vi "NACA0015_Polar.vi"() -> ()   [LabVIEW 2022 SP3]
panel:
  out "appended path":path
  in  "Stop Button":bool
  in  "Results folder":path
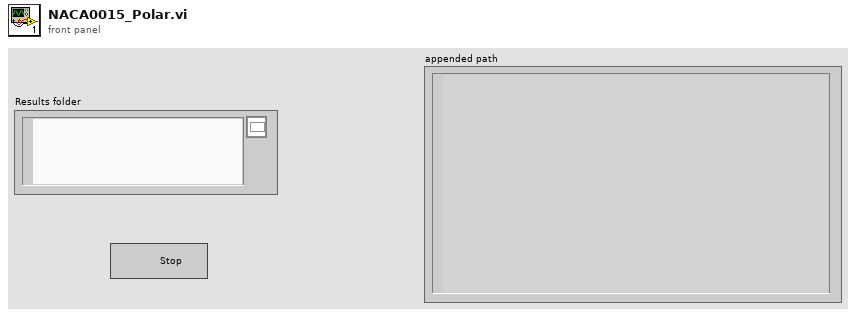
[diagram p1: front panel]
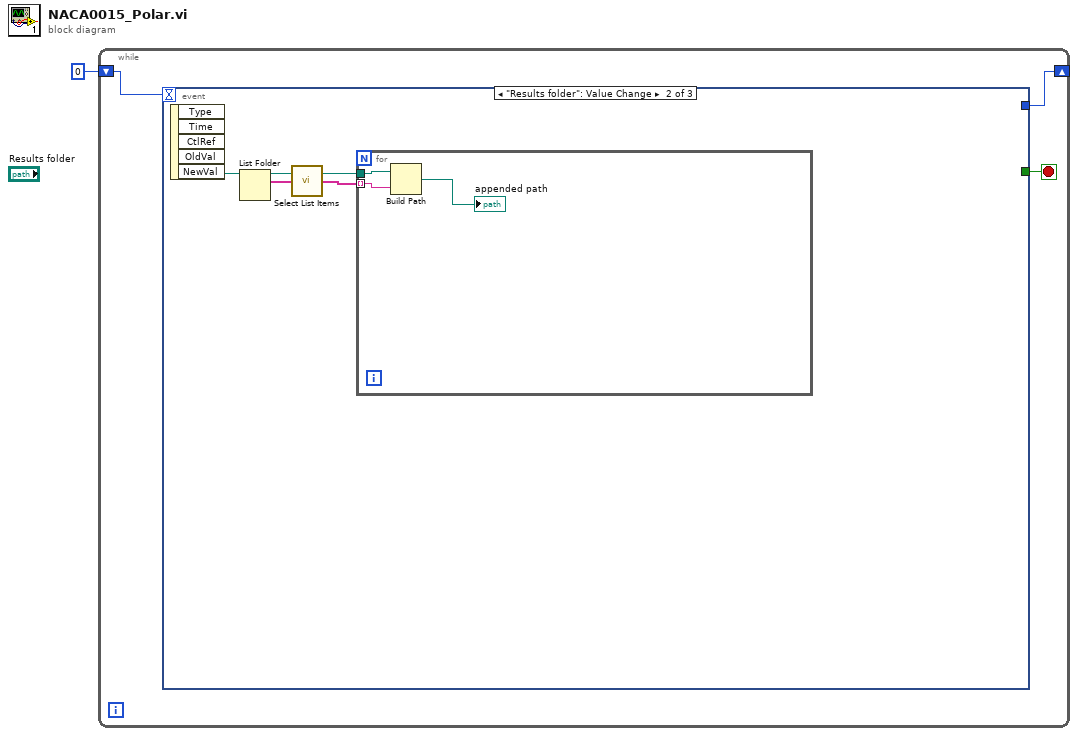
[diagram p0: block diagram]
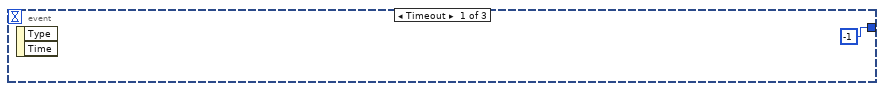
[diagram p2: hidden frame]
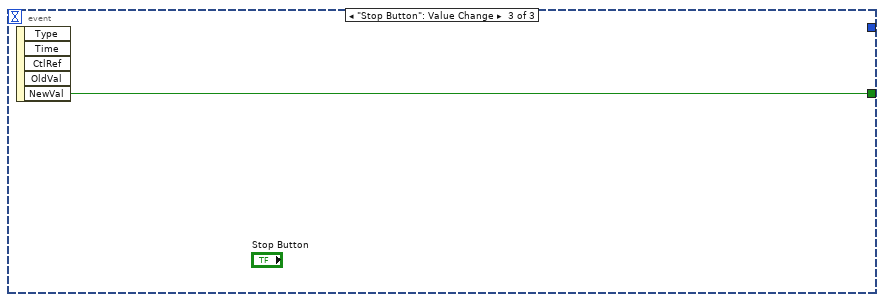
[diagram p3: hidden frame]
diagram:
  n1 = while {
    shift-right: [w3] -> _
    shift-left: 0 -> [w4]
    stop <- w2 stop-if-true
    n2 = event shown="[1] \"Results folder\": Value Change" {
      selector: _ -> [_ _ _]
      dyn-events: _ -> [_ _ _]
      timeout: w4 -> [_ _ _]
      tunnel: [-1 _ _] -> w3
      tunnel: [_ _ w13] -> w2
      event Timeout {
        n3 = event-data() -> ()  [unwired: 1 in, 2 out]
      }
      event "Results folder": Value Change {
        n4 = event-data() -> ("NewVal"=w6:path)  [unwired: 1 in, 4 out]
        n5 = List Folder(path=w6) -> (path out=w8:path, filenames=w9:string[])  [unwired: 3 in, 2 out]
        n6 = call "Select List Items.vi"("Item Names"=w9) -> ("Selected Items"=w7:string[])  [unwired: 4 in]
        n7 = for {
          tunnel: w8 -> [w12]
          tunnel: w7 -> [w11] mode=indexing
          n8 = Build Path(base path=w12, name or relative path=w11) -> (appended path=→"appended path":path)
        }
      }
      event "Stop Button": Value Change {
        n9 = event-data() -> ("NewVal"=w13:bool)  [unwired: 1 in, 4 out]
      }
    }
  }
